vi "Launcher.vi"   [LabVIEW 2012]
uses:
  Parent Actor/Parent Actor.lvclass
  <vilib>/ActorFramework/Message Queue/Message Queue.lvclass/Message Queue.ctl
  <vilib>/ActorFramework/Message Queue/Message Queue.lvclass
  <vilib>/ActorFramework/Actor/Actor.lvclass
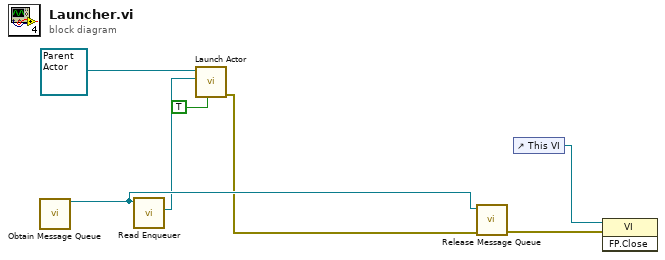
[diagram p0: block diagram]
diagram:
  n1 = call <vilib>:"Obtain Message Queue.vi"() -> ("Message Queue"=w7:refnum<class "Message Queue.lvclass">)  [unwired: 10 in, 1 out]
  n2 = call <vilib>:"Read Enqueuer.vi"("Message Queue"=w7) -> ("Message Enqueuer"=w5:refnum<class "Message Enqueuer.lvclass">)  [unwired: 10 in]
  n3 = call <vilib>:"Launch Actor.vi"("Open Actor Core front panel? (F)"=TRUE, "Actor-to-Caller Enqueuer"=w5, "Actor"=refnum<class "Parent Actor.lvclass"> refnum ("Parent Actor.lvclass")) -> ("error out"=w4:errorcluster)  [unwired: 7 in, 1 out]
  n4 = call <vilib>:"Release Message Queue.vi"("error in (no error)"=w4, "Message Queue"=w7) -> ("error out"=w1:errorcluster)  [unwired: 8 in, 1 out]
  n5 = control-ref of="This VI"() -> (w2:refnum<vi>)
  n6 = invoke class="VI" method="FP.Close"(reference=w2, error in=w1) -> ()  [unwired: 1 in, 3 out]
